vi "SPECAN_TXP_LOADPULL.vi"() -> ()   [LabVIEW 2016]
doc: "This example demonstrates how to use the Focus Microwaves tuner for an impedance sweep. This example measures the SpecAn transmission power (TxP) when the tuner moves to each impedance. The measurement results display on a Smith chart."
uses:
  <instrlib>/niRFSG/niRFSG.llb/niRFSG Exported Signal Destinations.ctl
  Source/SG/Typedefs/Instrument Configuration.ctl
  <instrlib>/niRFSG/niRFSG.llb/niRFSG Ref Clock Sources.ctl
  Source/Common/Local Oscillator Sharing Mode.ctl
  Source/Common/SA Common Configuration.ctl
  Source/SA/RFmxSpecAn/Typedefs/SpecAn TxP Configuration.ctl
  Source/SA/RFmxInstr/Typedefs/Instrument Configuration.ctl
  Source/Common/SA Auto Level Configuration.ctl
  Source/FocusTuner/Typedefs/Common Configuration.ctl
  Source/FocusTuner/Typedefs/S Parameters.ctl
  <userlib>/_RFIC Smith Chart/RFIC Smith Chart.xctl
  Source/SA/RFmxSpecAn/Typedefs/SpecAn TxP Results.ctl
  <vilib>/RFmx/SpecAn/mx/RFmxSpecAn.llb/RFmxSpecAn TXP Fetch Power Trace.vi
  Source/SG/SG.lvlib
  Source/SA/RFmxSpecAn/RFmxSpecAn.lvlib
  Source/SA/RFmxInstr/RFmxInstr.lvlib
  <instrlib>/Focus iTuner Series/Focus iTuner Series.lvlib
  Source/FocusTuner/FocusTuner.lvlib
  Source/Common/Common.lvlib
panel:
  in  "Display Tab Control":enum32{"Tuner Results", "TxP Results"}(tab)
  out "RFIC Smith Chart":cluster{"Gamma":cdb[], "Characteristic":dbl[]}(xcontrol)
  out "Primary Frequency (Hz)":dbl=3000000000.0 format="%_6p"
  out "Total Sweep Iterations":i32
  out "Current Sweep Iteration":i32
  out "TxP Results":T1[](array[typedef]) {"Minimum Power (dBm)" format="%.2f"; "Maximum Power (dBm)" format="%.2f"; "Peak to Average Ratio (dB)" format="%.2f"; "Average Mean Power (dBm)" format="%.2f"}
  out "Last Power Trace":cluster{"x0":dbl, "dx":dbl, "y":sgl[]}(graph)={"x0"=0.0, "dx"=3.999999999999943e-08, "y"=array[25000 elements]}
  in  "Measurement Settings Tab Control":enum32{"Tuner", "TxP"}(tab)
  in  "Sweep Type":enum32{"Constant VSWR", "Custom Sweep"}(tab)
  in  "Number of points":i32=20
  in  "VSWR":dbl=2.0 format="%#_13g"
  in  "Gamma Array":cdb[](array[numeric])=[0.6+0.0i, 0.596713137220964+0.06271707796059207i, 0.5868885604402834+0.12474701449065559i, 0.5706339097770922+0.18541019662496844i, 0.5481272745855605+0.2440419858454801i, 0.5196152422706631+0.29999999999999993i, 0.4854101966249684+0.3526711513754838i, 0.44588689528643655+0.40147836381531493i, 0.40147836381531493+0.4458868952864365i, 0.3526711513754839+0.4854101966249684i, 0.30000000000000004+0.5196152422706631i, 0.24404198584548023+0.5481272745855604i, 0.18541019662496847+0.5706339097770922i, 0.12474701449065555+0.5868885604402834i, 0.06271707796059207+0.596713137220964i, 3.6738190614671314e-17+0.6i, -0.06271707796059199+0.596713137220964i, -0.12474701449065546+0.5868885604402834i, -0.1854101966249684+0.5706339097770922i, -0.24404198584548004+0.5481272745855605i, -0.2999999999999999+0.5196152422706632i, -0.3526711513754838+0.4854101966249685i, -0.40147836381531476+0.44588689528643666i, -0.4458868952864366+0.4014783638153148i, -0.4854101966249684+0.35267115137548394i, -0.5196152422706631+0.3i, -0.5481272745855605+0.24404198584548i, -0.570633909777092+0.18541019662496852i, -0.5868885604402834+0.12474701449065558i, -0.596713137220964+0.06271707796059224i, -0.6+7.347638122934263e-17i, -0.596713137220964-0.06271707796059209i, -0.5868885604402834-0.12474701449065544i, -0.570633909777092-0.18541019662496863i, -0.5481272745855607-0.24404198584547987i, -0.5196152422706631-0.30000000000000004i, -0.4854101966249685-0.35267115137548377i, -0.44588689528643655-0.40147836381531493i, -0.40147836381531504-0.4458868952864364i, -0.35267115137548394-0.48541019662496837i, -0.3000000000000002-0.519615242270663i, -0.24404198584548004-0.5481272745855605i, -0.18541019662496855-0.570633909777092i, -0.12474701449065588-0.5868885604402833i, -0.06271707796059255-0.596713137220964i, -1.1021457184401395e-16-0.6i, 0.06271707796059232-0.596713137220964i, 0.12474701449065566-0.5868885604402834i, 0.18541019662496833-0.5706339097770922i, 0.24404198584547984-0.5481272745855607i, 0.30000000000000004-0.5196152422706631i, 0.35267115137548377-0.48541019662496854i, 0.4014783638153151-0.4458868952864364i, 0.4458868952864362-0.40147836381531526i, 0.48541019662496837-0.352671151375484i, 0.519615242270663-0.30000000000000027i, 0.5481272745855605-0.2440419858454801i, 0.570633909777092-0.18541019662496858i, 0.5868885604402833-0.12474701449065591i, 0.596713137220964-0.06271707796059257i, 0.5+0.0i, 0.49605735065723894+0.06266661678215213i, 0.48429158056431554+0.1243449435824274i, 0.46488824294412573+0.18406227634233896i, 0.4381533400219318+0.24087683705085766i, 0.4045084971874737+0.29389262614623657i, 0.3644843137107058+0.3422735529643443i, 0.3187119948743448+0.3852566213878946i, 0.2679133974894983+0.42216396275100754i, 0.21288964578253633+0.4524135262330098i, 0.15450849718747373+0.47552825814757677i, 0.09369065729286237+0.4911436253643443i, 0.03139525976465676+0.4990133642141358i, -0.0313952597646567+0.4990133642141358i, -0.09369065729286241+0.4911436253643443i, -0.15450849718747367+0.4755282581475768i, -0.21288964578253636+0.45241352623300973i, -0.26791339748949844+0.4221639627510075i, -0.3187119948743449+0.3852566213878946i, -0.36448431371070567+0.3422735529643444i, -0.40450849718747367+0.2938926261462366i, -0.4381533400219317+0.2408768370508578i, -0.4648882429441257+0.18406227634233907i, -0.48429158056431554+0.12434494358242741i, -0.4960573506572389+0.06266661678215227i, -0.5+6.123031769111886e-17i, -0.49605735065723894-0.06266661678215214i, -0.48429158056431554-0.12434494358242751i, -0.4648882429441256-0.18406227634233915i, -0.43815334002193185-0.2408768370508575i, -0.4045084971874738-0.2938926261462365i, -0.3644843137107058-0.34227355296434436i, -0.31871199487434476-0.3852566213878947i, -0.26791339748949816-0.42216396275100765i, -0.21288964578253608-0.4524135262330099i, -0.15450849718747378-0.47552825814757677i, -0.09369065729286231-0.49114362536434436i, -0.031395259764656604-0.4990133642141358i, 0.031395259764656416-0.4990133642141358i, 0.09369065729286213-0.49114362536434436i, 0.15450849718747361-0.4755282581475768i, 0.2128896457825359-0.45241352623300995i, 0.267913397489498-0.42216396275100776i, 0.31871199487434465-0.3852566213878948i, 0.3644843137107056-0.3422735529643445i, 0.40450849718747367-0.2938926261462367i, 0.4381533400219318-0.24087683705085766i, 0.46488824294412556-0.18406227634233935i, 0.4842915805643155-0.12434494358242767i, 0.4960573506572389-0.06266661678215232i, 0.4+0.0i, 0.39507533623805513+0.06257378601609234i, 0.3804226065180615+0.12360679774997897i, 0.35640260967534715+0.1815961998958187i, 0.32360679774997897+0.23511410091698925i, 0.282842712474619+0.282842712474619i, 0.23511410091698928+0.32360679774997897i, 0.18159619989581874+0.35640260967534715i, 0.123606797749979+0.3804226065180614i, 0.06257378601609237+0.39507533623805513i, 2.4492127076447546e-17+0.4i, -0.06257378601609241+0.39507533623805513i, -0.12360679774997894+0.3804226065180615i, -0.1815961998958187+0.3564026096753472i, -0.23511410091698923+0.323606797749979i, -0.282842712474619+0.28284271247461906i, -0.32360679774997897+0.23511410091698928i, -0.35640260967534715+0.18159619989581877i, -0.3804226065180614+0.12360679774997901i, -0.39507533623805513+0.0625737860160924i, -0.4+4.898425415289509e-17i, -0.39507533623805513-0.0625737860160923i, -0.3804226065180614-0.1236067977499791i, -0.35640260967534726-0.18159619989581852i, -0.323606797749979-0.23511410091698923i, -0.28284271247461906-0.282842712474619i, -0.2351141009169893-0.32360679774997897i, -0.1815961998958188-0.35640260967534715i, -0.12360679774997904-0.3804226065180614i, -0.06257378601609243-0.3950753362380551i, -7.347638122934264e-17-0.4i, 0.06257378601609227-0.39507533623805513i, 0.1236067977499789-0.3804226065180615i, 0.18159619989581866-0.3564026096753472i, 0.2351141009169892-0.323606797749979i, 0.28284271247461895-0.28284271247461906i, 0.3236067977499789-0.23511410091698934i, 0.35640260967534715-0.1815961998958188i, 0.3804226065180614-0.12360679774997907i, 0.3950753362380551-0.06257378601609244i, 0.3+0.0i, 0.2934442802201417+0.062373507245327794i, 0.27406363729278027+0.12202099292274005i, 0.2427050983124842+0.1763355756877419i, 0.20073918190765747+0.22294344764321825i, 0.15000000000000002+0.25980762113533157i, 0.09270509831248423+0.2853169548885461i, 0.03135853898029604+0.298356568610482i, -0.031358538980295995+0.298356568610482i, -0.0927050983124842+0.2853169548885461i, -0.14999999999999994+0.2598076211353316i, -0.20073918190765738+0.22294344764321833i, -0.2427050983124842+0.17633557568774197i, -0.27406363729278027+0.12202099292274i, -0.2934442802201417+0.06237350724532779i, -0.3+3.6738190614671314e-17i, -0.2934442802201417-0.06237350724532772i, -0.2740636372927803-0.12202099292273993i, -0.24270509831248424-0.17633557568774189i, -0.20073918190765752-0.2229434476432182i, -0.1500000000000001-0.2598076211353315i, -0.09270509831248427-0.285316954888546i, -0.03135853898029627-0.298356568610482i, 0.03135853898029616-0.298356568610482i, 0.09270509831248416-0.2853169548885461i, 0.15000000000000002-0.25980762113533157i, 0.20073918190765755-0.2229434476432182i, 0.24270509831248419-0.176335575687742i, 0.27406363729278027-0.12202099292274005i, 0.29344428022014163-0.062373507245327954i, 0.2+0.0i, 0.19021130325903074+0.061803398874989486i, 0.16180339887498948+0.11755705045849463i, 0.11755705045849464+0.16180339887498948i, 0.0618033988749895+0.1902113032590307i, 1.2246063538223773e-17+0.2i, -0.06180339887498947+0.19021130325903074i, -0.11755705045849461+0.1618033988749895i, -0.16180339887498948+0.11755705045849464i, -0.1902113032590307+0.06180339887498951i, -0.2+2.4492127076447546e-17i, -0.1902113032590307-0.06180339887498955i, -0.1618033988749895-0.11755705045849461i, -0.11755705045849466-0.16180339887498948i, -0.06180339887498952-0.1902113032590307i, -3.673819061467132e-17-0.2i, 0.06180339887498945-0.19021130325903074i, 0.1175570504584946-0.1618033988749895i, 0.16180339887498946-0.11755705045849467i, 0.1902113032590307-0.061803398874989535i, 0.1+0.0i, 0.08090169943749474+0.058778525229247314i, 0.03090169943749475+0.09510565162951536i, -0.030901699437494736+0.09510565162951537i, -0.08090169943749474+0.05877852522924732i, -0.1+1.2246063538223773e-17i, -0.08090169943749476-0.05877852522924731i, -0.03090169943749476-0.09510565162951536i, 0.030901699437494726-0.09510565162951537i, 0.08090169943749473-0.058778525229247335i, 0.0+0.0i]
  in  "IP Address":string="10.0.0.1"
  in  "Common Configuration":T2={"Tuner Mode"=1, "Calibration ID"=1, "DUT to Tuner S-parameters"=[{"S11"=0.0+0.0i, "S21"=1.0+0.0i, "S12"=1.0+0.0i, "S22"=0.0+0.0i}], "Load Termination"=[0.0+0.0i]} {"Tuner Mode" items=["Source", "Load"]}
  in  "TxP Configuration":T4={"Measurement Interval (s)"=0.001, "RBW (Hz)"=20000000.0, "RBW Filter Type"=5, "RRC Alpha"=0.0, "Averaging Enabled"=0, "Averaging Count"=10, "Averaging Type"=0} {"Averaging Type" items=["RMS", "Log", "Scalar", "Max", "Min"]; "Averaging Enabled" items=["False", "True"]; "RRC Alpha" format="%.3g"; "RBW Filter Type" items=["None"=5, "Gaussian"=1, "Flat"=2, "RRC"=6]; "RBW (Hz)" format="%.3p"; "Measurement Interval (s)" format="%.2p"}
  in  "Resource Control":enum32{"RFSG", "RFSA"}(tab)
  in  "Marker Event Output Terminal":T5="PXI_Trig0"
  in  "Reference Waveform File Path":path=path "C:/Users/Public/Documents/National Instruments/RFIC Test Software/Waveforms/LTE_FDD_UL_1x20MHz_256QAM_OS4.tdms"
  in  "RFSG Resource Name":refnum<k15>="5841"
  in  "SG Configuration":T6={"SelectedPorts"="", "Reference Clock Source"="PXI_CLK", "Carrier Frequency (Hz)"=3500000000.0, "DUT Average Input Power (dBm)"=-10.0, "External Attenuation (dB)"=0.0, "LO Sharing Mode"=enum."Automatic"}
  in  "RFSA Resource Name":refnum<k15>="5841"
  in  "RFmx SpecAn Configuration":T9={"Center Frequency (Hz)"=1000000000.0, "Reference Level (dBm)"=0.0, "External Attenuation (dB)"=0.0, "Trigger Enabled"=TRUE, "Digital Trigger Source"="PXI_Trig0", "Trigger Delay (s)"=0.0, "Selected Ports"=""} {"Trigger Delay (s)" format="%.2p"; "External Attenuation (dB)" format="%.2f"; "Reference Level (dBm)" format="%.2f"; "Center Frequency (Hz)" format="%.6p"}
  in  "Instrument Configuration":T10={"LO Sharing Mode"=enum."Automatic", "Frequency Reference Source"="PXI_Clk"}
  in  "Auto Level Configuration":T11={"Enabled"=TRUE, "Measurement Interval (s)"=0.01} {"Measurement Interval (s)" min=1e-06 max=100.0 format="%.2p"}
  in  "Auto Level Bandwidth (Hz)":dbl=20000000.0 format="%#_13p"
  in  "Center Frequency / SG IF (Hz)":dbl=3000000000.0 format="%.6p"
  in  "Error Tab Control":enum32{"Page 1", "Page 2"}(tab)
  out "error out":errorcluster
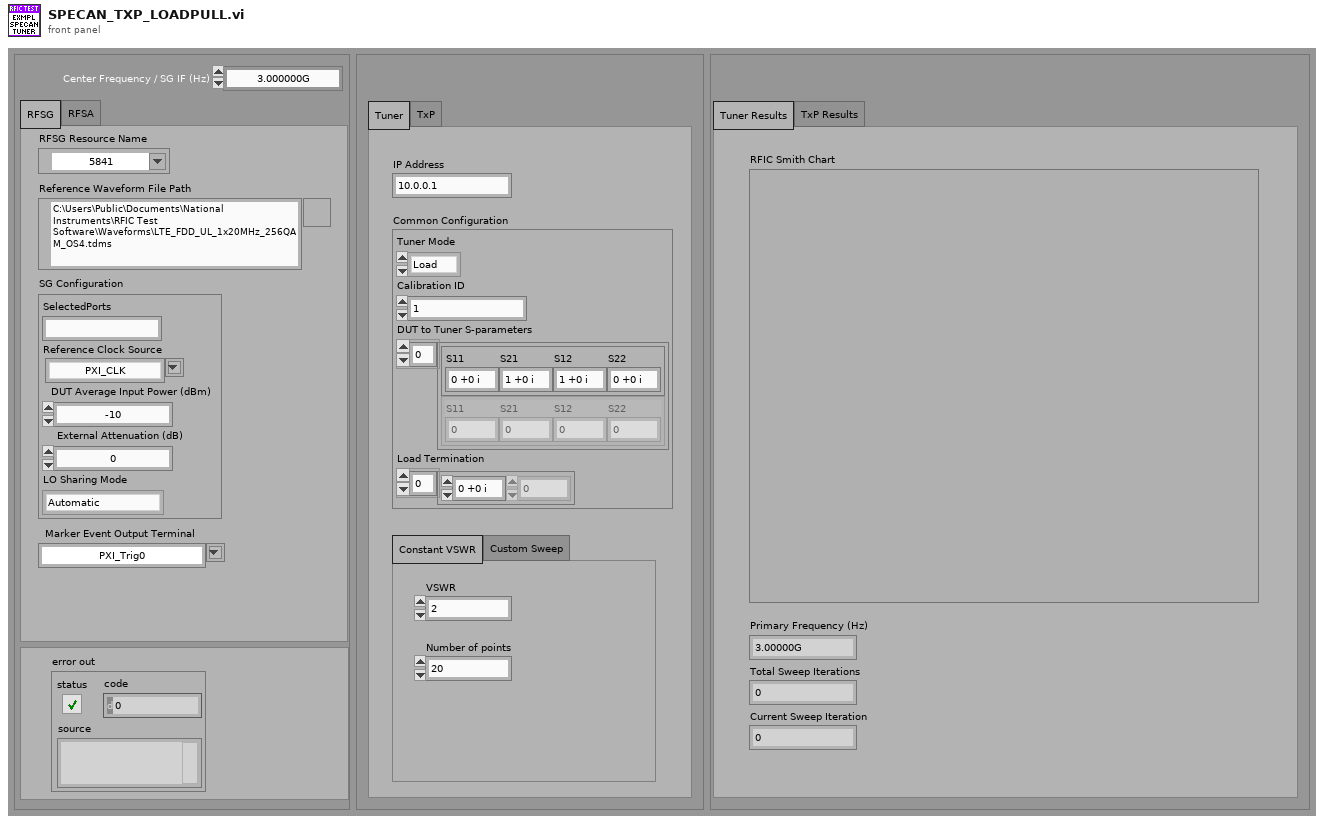
[diagram p1: front panel]
types:
  T1 = typedef "RFmxSpecAn.lvlib/SpecAn TxP Results.ctl" = cluster{"Average Mean Power (dBm)":dbl, "Peak to Average Ratio (dB)":dbl, "Maximum Power (dBm)":dbl, "Minimum Power (dBm)":dbl}
  T2 = typedef "FocusTuner.lvlib/Common Configuration.ctl" = cluster{"Tuner Mode":u16, "Calibration ID":i32, "DUT to Tuner S-parameters":T3[], "Load Termination":cdb[]}
  T3 = typedef "FocusTuner.lvlib/S Parameters.ctl" = cluster{"S11":cdb, "S21":cdb, "S12":cdb, "S22":cdb}
  T4 = typedef "RFmxSpecAn.lvlib/SpecAn TxP Configuration.ctl" = cluster{"Measurement Interval (s)":dbl, "RBW (Hz)":dbl, "RBW Filter Type":i32, "RRC Alpha":dbl, "Averaging Enabled":i32, "Averaging Count":i32, "Averaging Type":i32}
  T5 = typedef "niRFSG Exported Signal Destinations.ctl" = string
  T6 = typedef "SG.lvlib/Instrument Configuration.ctl" = cluster{"SelectedPorts":string, "Reference Clock Source":T7, "Carrier Frequency (Hz)":dbl, "DUT Average Input Power (dBm)":dbl, "External Attenuation (dB)":dbl, "LO Sharing Mode":T8}
  T7 = typedef "niRFSG Ref Clock Sources.ctl" = string
  T8 = typedef "Common.lvlib/Local Oscillator Sharing Mode.ctl" = enum16{"Automatic", "None"}
  T9 = typedef "Common.lvlib/SA Common Configuration.ctl" = cluster{"Center Frequency (Hz)":dbl, "Reference Level (dBm)":dbl, "External Attenuation (dB)":dbl, "Trigger Enabled":bool, "Digital Trigger Source":string, "Trigger Delay (s)":dbl, "Selected Ports":string}
  T10 = typedef "RFmxInstr.lvlib/Instrument Configuration.ctl" = cluster{"LO Sharing Mode":T8, "Frequency Reference Source":string}
  T11 = typedef "Common.lvlib/SA Auto Level Configuration.ctl" = cluster{"Enabled":bool, "Measurement Interval (s)":dbl}
  T12 = typedef "Common.lvlib/Waveform.ctl" = cluster{"Name":string, "Data":refnum<data-value>, "Signal Bandwidth (Hz)":dbl, "PAPR (dB)":dbl, "Burst Length (s)":dbl, "Sample Rate":dbl, "Burst Start Locations":i32[], "Burst Stop Locations":i32[], "Idle Duration Present?":bool, "Runtime Scaling":dbl, "Script":string}
  T13 = enum16{"ACP", "CCDF", "CHP", "FCnt", "Harmonics", "OBW", "SEM", "Spectrum", "Spur", "TXP", "AMPM", "DPD", "IQ", "IM", "NF", "PhaseNoise", "PAVT"}[]
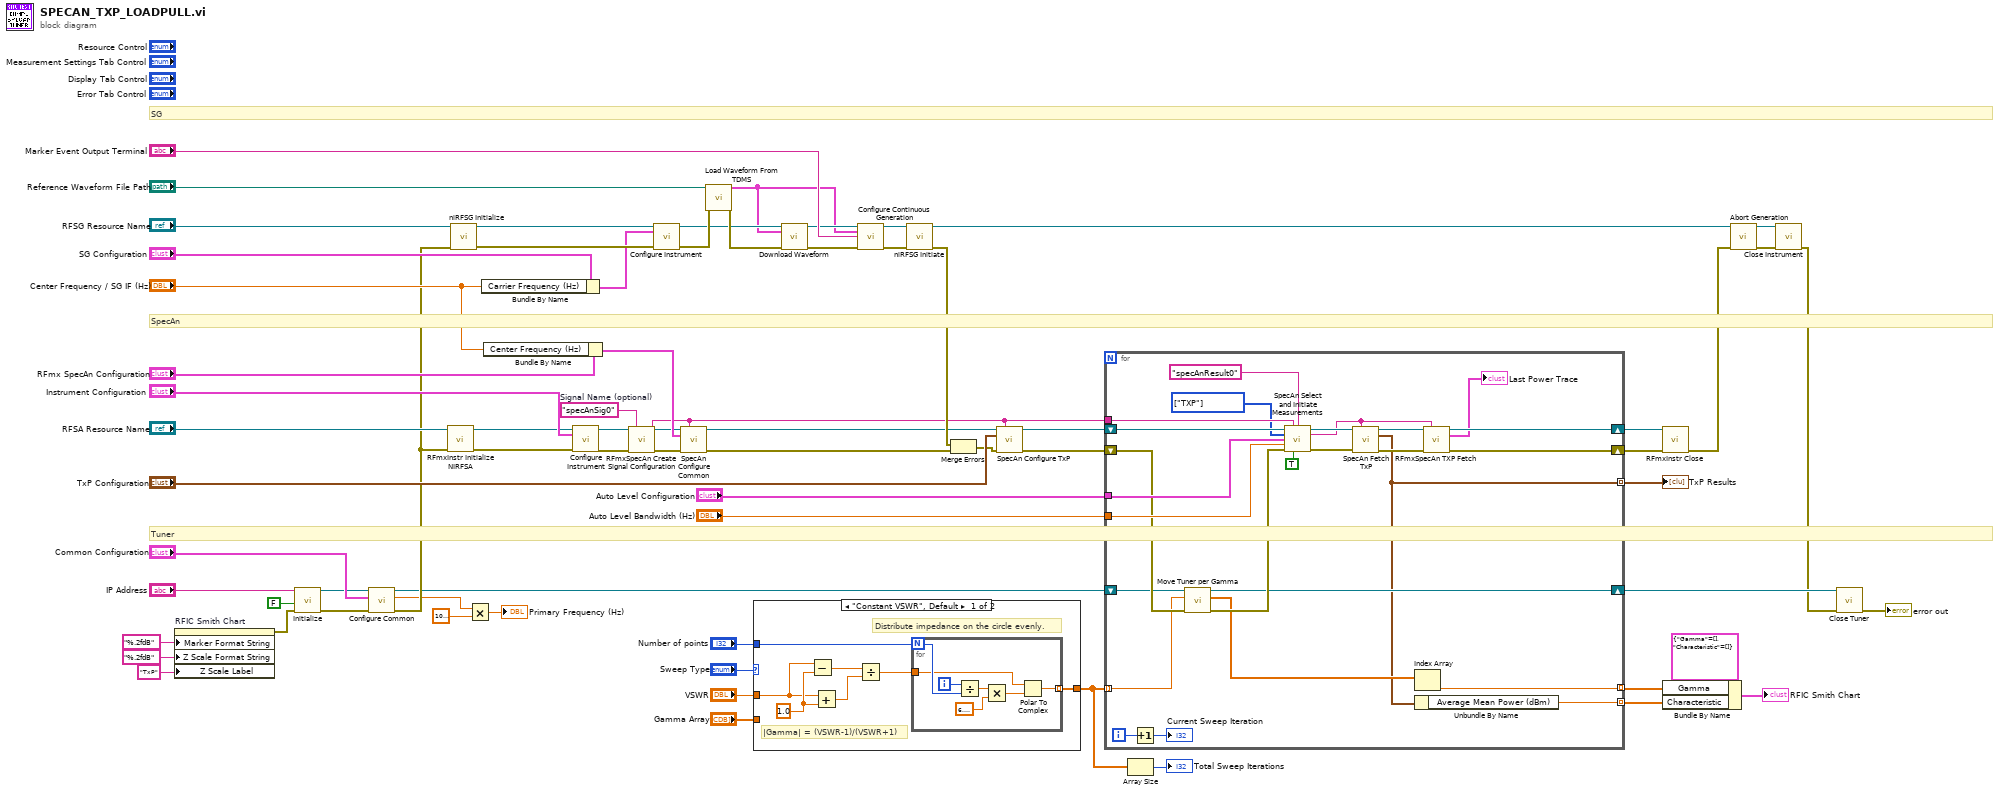
[diagram p0: block diagram]
diagram:
  w63 = "specAnSig0"  # Signal Name (optional)
  # "Tuner"
  # "SpecAn"
  # "SG"
  n1 = property on="RFIC Smith Chart" class="RFIC Smith Chart (strict)"("Marker Format String"="%.2fdB", "Z Scale Format String"="%.2fdB", "Z Scale Label"="TxP") -> (error out=w55:errorcluster)  [unwired: 2 in, 1 out]
  n2 = call <instrlib>:"Initialize.vi"("error in (no error)"=w55, "Reset (True)"=FALSE, "IP Address"="IP Address") -> ("error out"=w20:errorcluster, "iTuner reference out"=w21:refnum<k7>)  [unwired: 7 in]
  n3 = call "Configure Common.vi"("error in (no error)"=w20, "Common Configuration"="Common Configuration", "iTuner reference in"=w21) -> ("error out"=w26:errorcluster, "Primary Frequency (GHz)"=w5:dbl, "iTuner reference out"=w18:refnum<k7>)  [unwired: 6 in]
  n4 = call <vilib>:"RFmxInstr Initialize NIRFSA.vi"("Resource Name"="RFSA Resource Name", "error in (no error)"=w26) -> ("Instrument Handle Out"=w37:refnum<k21>, "error out"=w36:errorcluster)  [unwired: 11 in, 1 out]
  n5 = call <instrlib>:"niRFSG Initialize.vi"("resource name"="RFSG Resource Name", "error in"=w26) -> ("instrument handle"=w49:refnum<k15>, "error out"=w48:errorcluster)  [unwired: 12 in]
  n6 = Multiply(x=w5, y=1000000000.0) -> (x*y=→"Primary Frequency (Hz)":dbl)
  n7 = Bundle By Name(cluster="SG Configuration", "Carrier Frequency (Hz)"="Center Frequency / SG IF (Hz)") -> (w43:T6)
  n8 = Bundle By Name(cluster="RFmx SpecAn Configuration", "Center Frequency (Hz)"="Center Frequency / SG IF (Hz)") -> (w42:T9)
  n9 = call "Configure Instrument.vi"("Instrument Handle In"=w37, "Instrument Configuration"="Instrument Configuration", "error in (no error)"=w36) -> ("Instrument Handle Out"=w34:refnum<k21>, "error out"=w31:errorcluster)  [unwired: 11 in]
  n10 = call <vilib>:"RFmxSpecAn Create Signal Configuration.vi"("Instrument Handle In"=w34, "Signal Name"=w63, "error in (no error)"=w31) -> ("Instrument Handle Out"=w33:refnum<k21>, "Selector String Out"=w32:string, "error out"=w30:errorcluster)  [unwired: 10 in]
  n11 = call "Configure Instrument.vi"("RFSG Session In"=w49, "SG Configuration"=w43, "error in (no error)"=w48) -> ("RFSG Session Out"=w52:refnum<k15>, "error out"=w54:errorcluster)  [unwired: 11 in]
  n12 = call "SpecAn Configure Common.vi"("RFmx Handle In"=w33, "Selector String"=w32, "Common Configuration"=w42, "error in (no error)"=w30) -> ("RFmx Handle Out"=w27:refnum<k21>, "error out"=w29:errorcluster)  [unwired: 10 in]
  n13 = call "Load Waveform From TDMS.vi"("TDMS File Path"="Reference Waveform File Path", "error in (no error)"=w54) -> ("Waveform"=w28:T12, "error out"=w53:errorcluster)  [unwired: 12 in]
  n14 = case shown="\"Constant VSWR\", Default" "Sweep Type" {
    tunnel: [w74 w86] -> w4
    tunnel: "Number of points" -> [w73 _]
    tunnel: "VSWR" -> [w72 _]
    tunnel: "Gamma Array" -> [_ w86]
    frame "Constant VSWR", Default {
      w78 = 1.0 ("y")
      # "Distribute impedance on the circle evenly."
      # "|Gamma| = (VSWR-1)/(VSWR+1)"
      n15 = Subtract(x=w72, y=w78) -> (x-y=w77:dbl)
      n16 = Add(x=w72, y=w78) -> (x+y=w76:dbl)
      n17 = Divide(x=w77, y=w76) -> (x/y=w75:dbl)
      n18 = for {
        N: w73 -> [w82]
        tunnel: [w84] -> w74 mode=indexing
        tunnel: w75 -> [w80]
        i -> [w83]
        n19 = Divide(x=w83, y=w82) -> (x/y=w81:dbl)
        n20 = Multiply(x=w81, y=6.283185307179586) -> (x*y=w79:dbl)
        n21 = Polar To Complex(1:w79, 2:w80) -> (0:w84:cdb)
      }
    }
    frame "Custom Sweep" {
    }
  }
  n22 = call "Download Waveform.vi"("RFSG handle"=w52, "Waveform In"=w28, "error in (no error)"=w53) -> ("RFSG handle out"=w47:refnum<k15>, "error out"=w45:errorcluster)  [unwired: 11 in]
  n23 = call "Configure Continuous Generation.vi"("RFSG handle"=w47, "Waveform in"=w28, "Waveform Start Trigger Export"="Marker Event Output Terminal", "error in"=w45) -> ("RFSG handle out"=w46:refnum<k15>, "error out"=w38:errorcluster)  [unwired: 9 in, 1 out]
  n24 = call <instrlib>:"niRFSG Initiate.vi"("instrument handle"=w46, "error in"=w38) -> ("instrument handle out"=w39:refnum<k15>, "error out"=w35:errorcluster)  [unwired: 12 in]
  n25 = Merge Errors(w35, w29) -> (w22:errorcluster)
  n26 = call "SpecAn Configure TxP.vi"("Instrument Handle In"=w27, "Selector String"=w32, "TxP Config"="TxP Configuration", "error in (no error)"=w22) -> ("Instrument Handle Out"=w23:refnum<k21>, "error out"=w19:errorcluster)  [unwired: 10 in]
  n27 = for {
    tunnel: w32 -> [w110]
    tunnel: "Auto Level Bandwidth (Hz)" -> [w109]
    tunnel: "Auto Level Configuration" -> [w108]
    shift-right: [w112] -> w41
    shift-left: w23 -> [w104]
    shift-right: [w111] -> w40
    shift-left: w19 -> [w96]
    shift-right: [w94] -> w17
    shift-left: w18 -> [w95]
    tunnel: w4 -> [w93] mode=indexing
    tunnel: [w91] -> w13 mode=indexing
    tunnel: [w90] -> w11 mode=indexing
    tunnel: [w89] -> w10 mode=indexing
    i -> [w88]
    w101 = T13 [enum."TXP"] items=["ACP", "CCDF", "CHP", "FCnt", "Harmonics", "OBW", "SEM", "Spectrum", "Spur", "TXP", "AMPM", "DPD", "IQ", "IM", "NF", "PhaseNoise", "PAVT"] ("Measurements")
    n28 = Increment(x=w88) -> (x+1=→"Current Sweep Iteration":i32)
    n29 = call "Move Tuner per Gamma.vi"("error in (no error)"=w96, "Gamma"=w93, "iTuner reference in"=w95) -> ("error out"=w97:errorcluster, "Current Gammas"=w92:cdb[], "iTuner reference out"=w94:refnum<k7>)  [unwired: 6 in]
    n30 = call "SpecAn Select and Initiate Measurements.vi"("Instrument Handle In"=w104, "Selector String"=w110, "Result Name"="specAnResult0", "Measurements"=w101, "Auto Level Configuration"=w108, "Auto Level Bandwidth (Hz)"=w109, "error in (no error)"=w97, "Enable All Traces (F)"=TRUE) -> ("Instrument Handle Out"=w103:refnum<k21>, "Selector String Out"=w99:string, "error out"=w102:errorcluster)  [unwired: 5 in]
    n31 = call "SpecAn Fetch TxP.vi"("Instrument Handle In"=w103, "Selector String"=w99, "error in (no error)"=w102) -> ("Instrument Handle Out"=w107:refnum<k21>, "TxP Results"=w91:T1, "error out"=w106:errorcluster)  [unwired: 10 in]
    n32 = Index Array(array=w92) -> (element=w90:cdb)  [unwired: 1 in]
    n33 = Unbundle By Name(w91) -> ("Average Mean Power (dBm)"=w89:dbl)
    n34 = call-poly <vilib>:"RFmxSpecAn TXP Fetch.vi"("Instrument Handle In"=w107, "Selector String"=w99, "error in (no error)"=w106) -> ("Instrument Handle Out"=w112:refnum<k21>, "Power (dBm)"=→"Last Power Trace":cluster{"x0":dbl, "dx":dbl, "y":sgl[]}, "error out"=w111:errorcluster)  [unwired: 10 in]
  }
  "TxP Results" <- w13
  n35 = Array Size(array=w4) -> (size(s)=→"Total Sweep Iterations":i32)
  n36 = call <vilib>:"RFmxInstr Close.vi"("Instrument Handle In"=w41, "error in (no error)"=w40) -> ("error out"=w44:errorcluster)  [unwired: 13 in]
  n37 = Bundle By Name(cluster=cluster{"Gamma":cdb[], "Characteristic":dbl[]} {"Gamma"=[], "Characteristic"=[]} ("Single Point"), "Gamma"=w11, "Characteristic"=w10) -> (→"RFIC Smith Chart":cluster{"Gamma":cdb[], "Characteristic":dbl[]})
  n38 = call "Abort Generation.vi"("RFSG handle"=w39, "error in (no error)"=w44) -> ("RFSG handle out"=w51:refnum<k15>, "error out"=w50:errorcluster)  [unwired: 12 in]
  n39 = call "Close Instrument.vi"("RFSG Handle"=w51, "error in (no error)"=w50) -> ("error out"=w16:errorcluster)  [unwired: 13 in]
  n40 = call "Close Tuner.vi"("error in (no error)"=w16, "iTuner reference in"=w17) -> ("error out"=→"error out":errorcluster)  [unwired: 9 in]
